vi "Swap X and Y (multiple).vi"(8 "error in (no error)":errorcluster, 11 "XY-data":cluster{"X-array":dbl[], "Y-array":dbl[]}[](array[cluster]) {"Y-array" format="%.2p"; "X-array" format="%.2p"}) -> (0 "error out":errorcluster, 3 "XY-data out":cluster{"X-array":dbl[], "Y-array":dbl[]}[](array[cluster]) {"Y-array" format="%.2p"; "X-array" format="%.2p"})   [LabVIEW 2019, in "xy_utilities.lvlib"]
doc: "Swap the x and y arrays.\n\nWire data to the data input to determine the polymorphic instance to use or manually select the instance."
uses:
  xy_utilities.lvlib
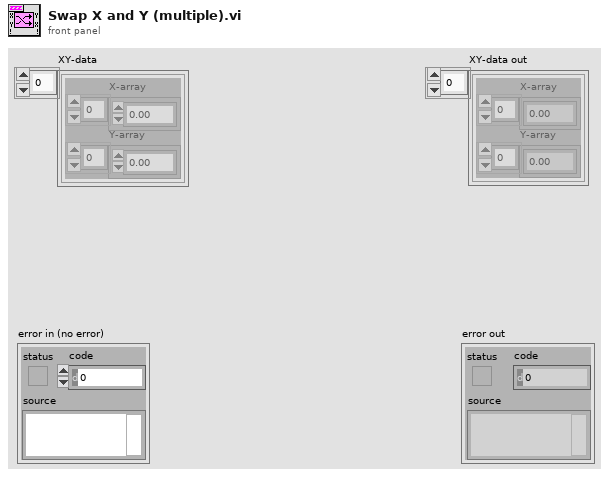
[diagram p1: front panel]
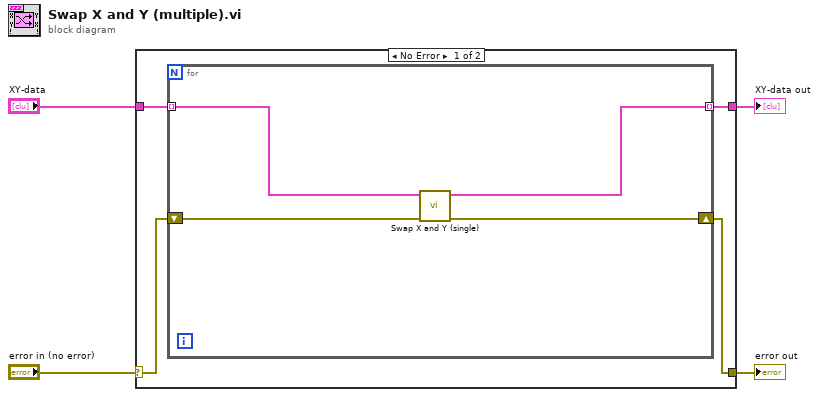
[diagram p0: block diagram]
diagram:
  n1 = case shown="No Error" "error in (no error)" {
    selector: "error in (no error)" -> [w6 w14]
    tunnel: "XY-data" -> [w8 w13]
    tunnel: [w7 w13] -> w2
    tunnel: [w5 w14] -> w1
    frame No Error {
      n2 = for {
        tunnel: w8 -> [w12] mode=indexing
        tunnel: [w11] -> w7 mode=indexing
        shift-right: [w9] -> w5
        shift-left: w6 -> [w10]
        n3 = call "Swap X and Y (single).vi"("error in (no error)"=w10, "XY-data"=w12) -> ("error out"=w9:errorcluster, "XY-data out"=w11:cluster{"X-array":dbl[], "Y-array":dbl[]})  [unwired: 8 in]
      }
    }
    frame Error {
    }
  }
  "error out" <- w1
  "XY-data out" <- w2
